vi "testHF.vi"() -> ()   [LabVIEW 2019]
uses:
  modbusrtu/MB error message.ctl
  modbusrtu/Pick MB port.ctl
  modbusrtu/MB Director.ctl
  modbusrtu/MB cmd buffer.ctl
  Process Controller 3.0/Distributed Daq/Data cmd.ctl
  calibration/Shared Data/share data command.ctl
panel:
  out "error out":errorcluster
  out "Set Point names":string[](array[string])=["data interval (s)", "device ID"]
  out "quitting":bool
  out "MB Quit":bool
  out "ProCoDA message":string
  in  "Pick MB port":T1
  out "MB errors":T2[](array[typedef])
  out "relative seconds":dbl
  in  "Turb 2":bool
  out "output value 2":dbl
  in  "Turb 2":dbl[](array[numeric])=[1.0, 5.0]
  in  "Turb 1":bool
  out "output value 1":dbl
  in  "MTOL 1":dbl[](array[numeric])=[1.0, 10.0]
  in  "State":i16
  out "read in seconds":dbl
  out "Numeric":i32
  in  "stop":bool
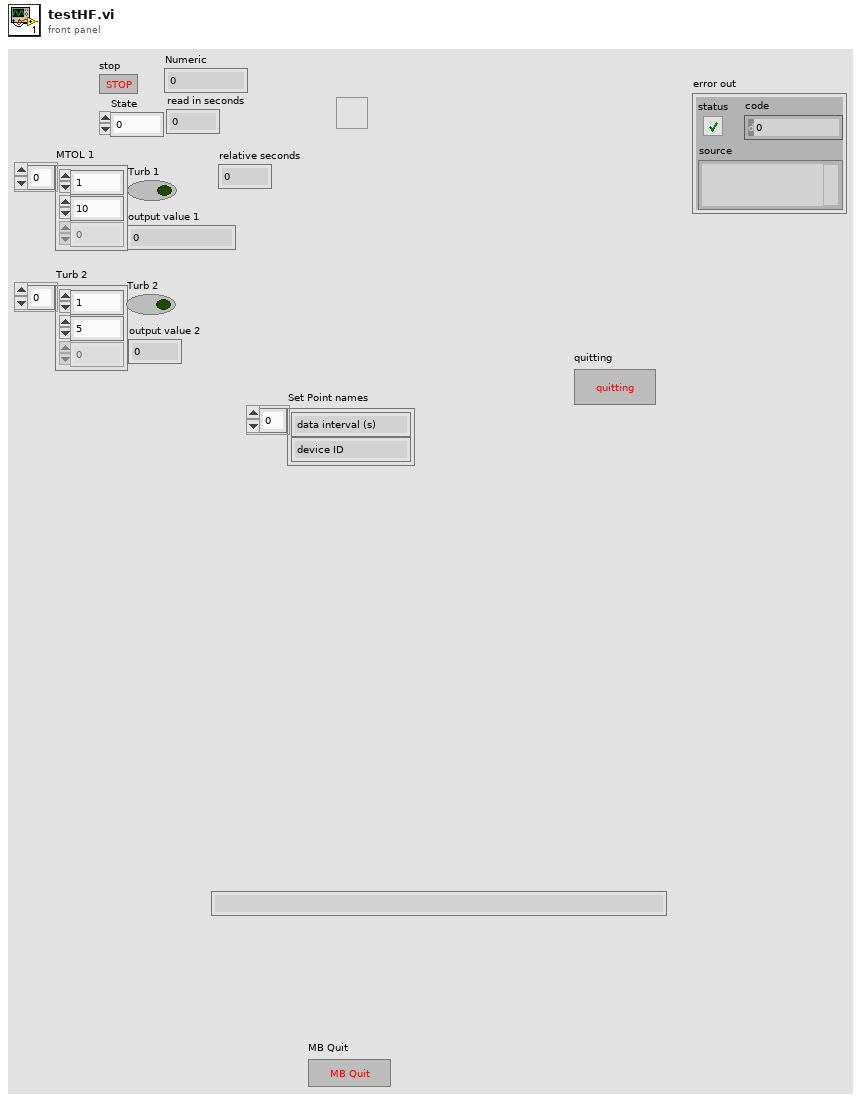
[diagram p1: front panel]
types:
  T1 = typedef "Pick MB port.ctl" = bool
  T2 = typedef "MB error message.ctl" = cluster{"message":string, "Device ID":u16}
  T3 = typedef "MB cmd buffer.ctl" = enum16{"ProCoDA", "MB succeed", "MB error", "MB Next Task", "ProCoDA read 1", "Commands pending"}
  T4 = typedef "MB Director.ctl" = enum16{"Config MB Port", "Run MB", "Get MB Port", "Quit MB"}
  T5 = typedef "share data command.ctl" = enum16{"Initialize from ini", "Update ini", "Write data", "Read data", "List my data", "List shared data", "Close"}
  T6 = typedef "Data cmd.ctl" = enum16{"User config", "Ini config", "Read Data", "Close"}
  T7 = enum32{"invalid app kind", "Development System", "Run Time System", "Student Edition", "Embedded LabVIEW", "Evaluation", "Custom"}
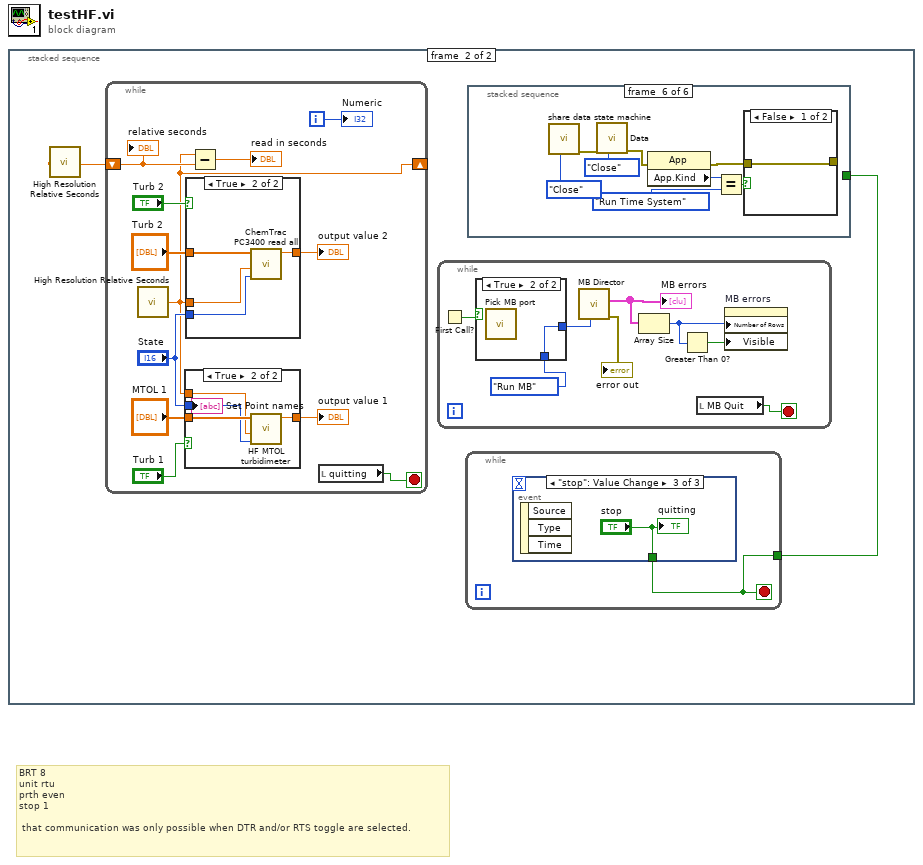
[diagram p0: block diagram]
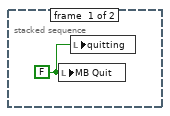
[diagram p2: hidden frame]
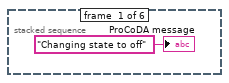
[diagram p3: hidden frame]
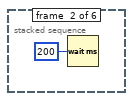
[diagram p4: hidden frame]
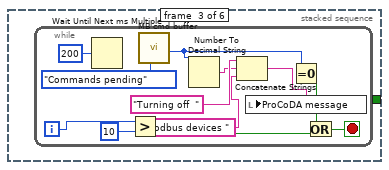
[diagram p5: hidden frame]
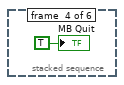
[diagram p6: hidden frame]
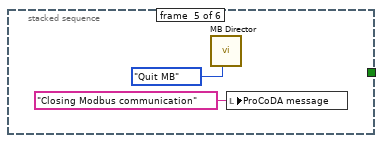
[diagram p7: hidden frame]
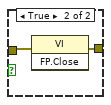
[diagram p8: hidden frame]
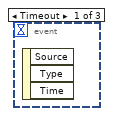
[diagram p9: hidden frame]
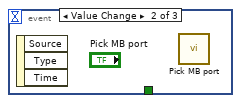
[diagram p10: hidden frame]
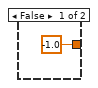
[diagram p12: hidden frame]
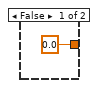
[diagram p13: hidden frame]
diagram:
  # "BRT 8\nunit rtu\nprth even\nstop 1\n\n that communication was only possible when DTR and/or RTS toggle are selected."
  n1 = stacked-sequence {
    frame #0 {
      w1 = FALSE ("MB Quit")
      n2 = local write "MB Quit"(w1) -> ()
      n3 = local write "quitting"(w1) -> ()
    }
    frame #1 {
      n4 = call <vilib>:"High Resolution Relative Seconds.vi"() -> ("relative seconds"=w3:dbl)
      n5 = while {
        shift-right: [w45] -> _
        shift-left: w3 -> [w55]
        i -> [w54]
        stop <- w44 stop-if-true
        n6 = call <vilib>:"High Resolution Relative Seconds.vi"() -> ("relative seconds"=w45:dbl)
        n7 = case shown="True" "Turb 1" {
          tunnel: "State" -> [_ w62]
          tunnel: [0.0 ("output value") w65] -> w52
          tunnel: "MTOL 1" -> [_ w64]
          tunnel: w45 -> [_ w63]
          frame False {
          }
          frame True {
            n8 = call "HF MTOL turbidimeter.vi"("State"=w62, "Time"=w63, "Set Points"=w64) -> ("output value"=w65:dbl)  [unwired: 3 in, 1 out]
          }
        }
        "output value 1" <- w52
        n9 = case shown="True" "Turb 2" {
          tunnel: "State" -> [_ w60]
          tunnel: "Turb 2" -> [_ w59]
          tunnel: w45 -> [_ w58]
          tunnel: [-1.0 ("output value") w57] -> w47
          frame False {
          }
          frame True {
            n10 = call "ChemTrac PC3400 read all.vi"("State"=w60, "Time"=w58, "Set Points"=w59) -> ("output value"=w57:dbl)  [unwired: 3 in, 1 out]
          }
        }
        "output value 2" <- w47
        n11 = Subtract(x=w45, y=w55) -> (x-y=→"read in seconds":dbl)
        n12 = local read "quitting"() -> (w44:bool)
        "Numeric" <- w54
        "relative seconds" <- w55
      }
      n13 = while {
        stop <- w38 stop-if-true
        n14 = First Call?() -> (First Call?: T/F=w37:bool)
        n15 = case shown="True" w37 {
          tunnel: [w42 w43] -> w36
          tunnel: MB_Director."Run MB" ("MB Director") -> [w42 w43]
          frame False {
          }
          frame True {
            n16 = call "Pick MB port.vi"() -> ()  [unwired: 12 in]
          }
        }
        n17 = call "MB Director.vi"("MB Director"=w36) -> ("error out"=→"error out":errorcluster, "MB errors"=w41:T2[])  [unwired: 8 in, 1 out]
        "MB errors" <- w41
        n18 = Array Size(array=w41) -> (size(s)=w40:i32)
        n19 = Greater Than 0?(x=w40) -> (x > 0?=w39:bool)
        n20 = local read "MB Quit"() -> (w38:bool)
        n21 = property on="MB errors" class="Arr (strict)"("Number of Rows"=w40, "Visible"=w39) -> ()  [unwired: 2 in, 2 out]
      }
      n22 = while {
        tunnel: [w32] -> w2
        stop <- w32 stop-if-true
        n23 = event shown="[2] \"stop\": Value Change" {
          selector: _ -> [_ _ _]
          dyn-events: _ -> [_ _ _]
          timeout: _ -> [_ _ _]
          tunnel: [_ _ "stop"] -> w32
          event Timeout {
            n24 = event-data() -> ()  [unwired: 1 in, 3 out]
          }
          event Value Change {
            n25 = event-data() -> ()  [unwired: 1 in, 3 out]
            n26 = call "Pick MB port.vi"() -> ()  [unwired: 12 in]
          }
          event "stop": Value Change {
            n27 = event-data() -> ()  [unwired: 1 in, 3 out]
            "quitting" <- "stop"
          }
        }
      }
      n28 = stacked-sequence {
        tunnel: w2 -> [_ _ _ _ _ _]
        frame #0 {
          "ProCoDA message" <- "Changing state to off" ("ProCoDA message")
        }
        frame #1 {
          n29 = Wait (ms)(milliseconds to wait=u32 200) -> ()  [unwired: 1 out]
        }
        frame #2 {
          n30 = while {
            i -> [w15]
            stop <- w11 stop-if-true
            n31 = Wait Until Next ms Multiple(millisecond multiple=u32 200) -> ()  [unwired: 1 out]
            n32 = Greater?(x=w15, y=10) -> (0:w12:bool)
            n33 = call "MB cmd buffer.vi"("MB cmd buffer"=MB_cmd_buffer."Commands pending") -> ("cmds pending"=w10:i16)  [unwired: 4 in, 6 out]
            n34 = Number To Decimal String(number=w10) -> (decimal integer string=w8:string)  [unwired: 1 in]
            n35 = Concatenate Strings("Turning off  " ("ProCoDA message"), w8, " modbus devices " ("ProCoDA message")) -> (w6:string)
            n36 = local write "ProCoDA message"(w6) -> ()
            n37 = Equal To 0?(x=w10) -> (x = 0?=w13:bool)
            n38 = Or(x=w13, y=w12) -> (x .or. y?=w11:bool)
          }
        }
        frame #3 {
          "MB Quit" <- TRUE ("MB Quit")
        }
        frame #4 {
          n39 = call "MB Director.vi"("MB Director"=MB_Director."Quit MB") -> ()  [unwired: 8 in, 3 out]
          n40 = local write "ProCoDA message"("Closing Modbus communication" ("ProCoDA message")) -> ()
        }
        frame #5 {
          n41 = call "share data state machine.vi"("Share data command"=share_data_command."Close") -> ("error out"=w21:errorcluster)  [unwired: 4 in, 6 out]
          n42 = call "Data.vi"("Data Command"=Data_cmd."Close", "error in"=w21) -> ("error out"=w23:errorcluster)  [unwired: 6 in, 3 out]
          n43 = property class="App"(error in=w23) -> (error out=w28:errorcluster, "App.Kind"=w26:T7)  [unwired: 1 in, 1 out]
          n44 = Equal?(x=w26, y=T7."Run Time System" ("Application:Kind")) -> (x = y?=w27:bool)
          n45 = case shown="False" w27 {
            tunnel: w28 -> [w29 w31]
            tunnel: [w29 w30] -> _
            frame False {
            }
            frame True {
              n46 = invoke class="VI" method="FP.Close"(error in=w31) -> (error out=w30:errorcluster)  [unwired: 2 in, 2 out]
            }
          }
        }
      }
    }
  }
